vi "GeneratePhaseGPU.vi"() -> ()   [LabVIEW 2019]
uses:
  <vilib>/vision/NI_Vision_Development_Module.lvlib
panel:
  in  "N Iterations":i32
  out "N Pixels":i32
  out "SLM Size":i32
  out "startCuda Return":i32
  in  "CUDA":bool
  out "stopCUDA Return":i32
  out "generatePhase Return":i32
  out "Path to Image File":path
  out "Desired Amplitude":sgl[][](array[numeric])
  in  "Update":bool
  out "Path to CUDA DLL":path
  out "Desired Amplitude":T1(plugin-control)
  in  "Stop":bool
  out "Phase SLM":T1(plugin-control)
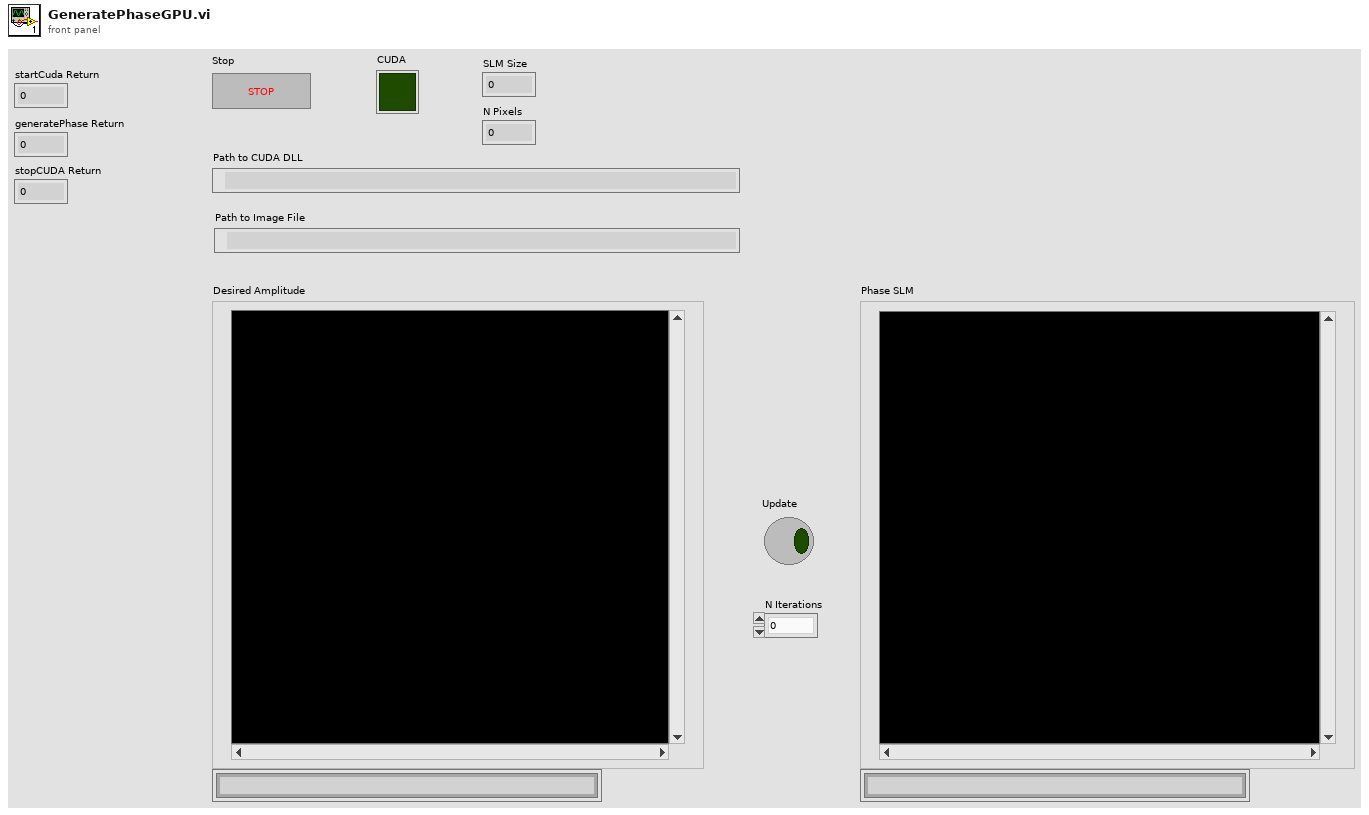
[diagram p1: front panel]
types:
  T1 = typedef "IMAQ Image.ctl" = refnum<image>
  T2 = typedef "Image Type" = u32
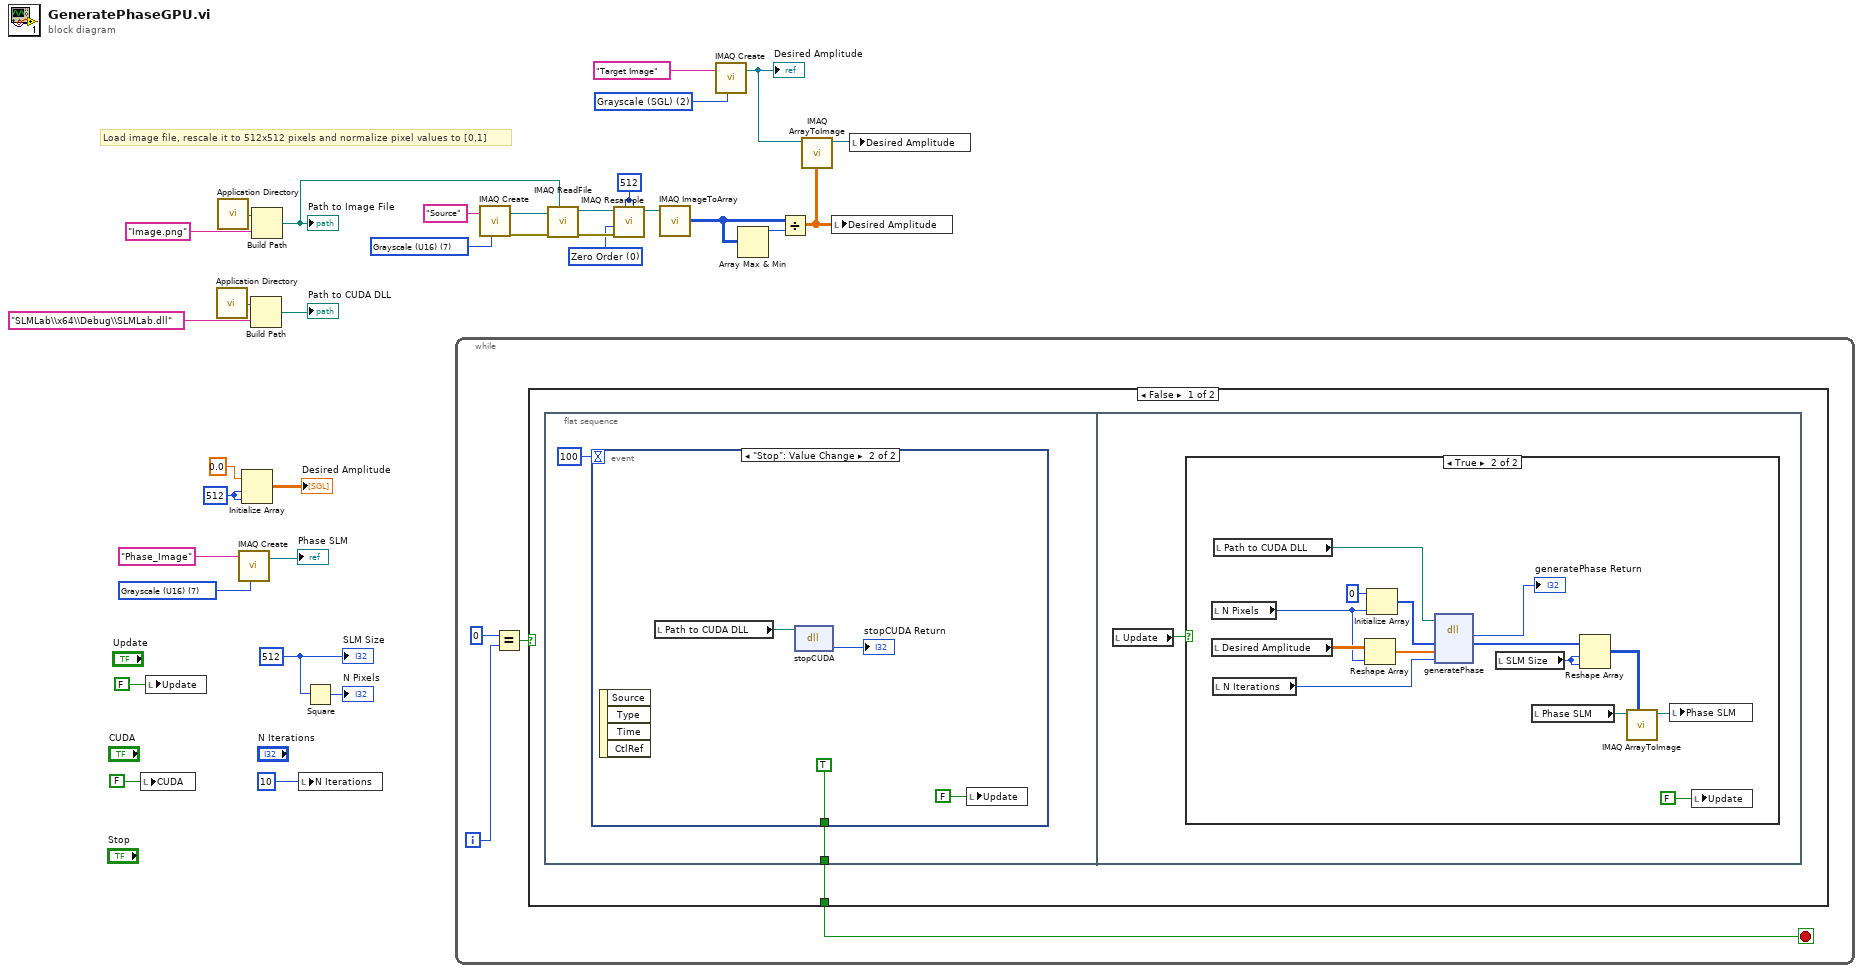
[diagram p0: block diagram]
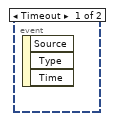
[diagram p2: hidden frame]
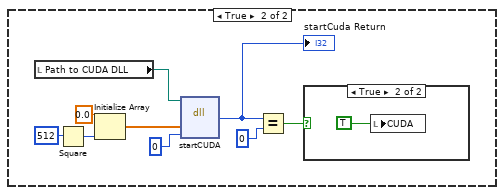
[diagram p4: hidden frame]
diagram:
  w3 = 512
  w16 = T2 7 items=["Grayscale (U8)", "Grayscale (I16)", "Grayscale (SGL)", "Complex (CSG)", "RGB (U32)", "HSL (U32)", "RGB (U64)", "Grayscale (U16)"] ("Image Type")
  w13 = 512
  w12 = u32 0 items=["Zero Order", "Bi-Linear", "Quadratic", "Cubic Spline"] ("Interpolation Type")
  w23 = 512 ("dimension size")
  w29 = T2 2 items=["Grayscale (U8)", "Grayscale (I16)", "Grayscale (SGL)", "Complex (CSG)", "RGB (U32)", "HSL (U32)", "RGB (U64)", "Grayscale (U16)"] ("Image Type")
  w32 = T2 7 items=["Grayscale (U8)", "Grayscale (I16)", "Grayscale (SGL)", "Complex (CSG)", "RGB (U32)", "HSL (U32)", "RGB (U64)", "Grayscale (U16)"] ("Image Type")
  # "Load image file, rescale it to 512x512 pixels and normalize pixel values to [0,1]"
  n1 = local write "CUDA"(FALSE ("Update SLM")) -> ()
  n2 = local write "Update"(FALSE ("Update SLM")) -> ()
  n3 = call <vilib>:"Application Directory.vi"() -> ("Application Directory"=w26:path)
  n4 = call <vilib>:"Application Directory.vi"() -> ("Application Directory"=w8:path)
  n5 = call "IMAQ Create"("Image Name"="Phase_Image", "Image Type"=w32) -> ("New Image"=→"Phase SLM":T1)  [unwired: 3 in, 1 out]
  n6 = Initialize Array(sgl 0.0, w23, w23) -> (→"Desired Amplitude":sgl[][])
  n7 = Build Path(base path=w26, name or relative path="SLMLab\\x64\\Debug\\SLMLab.dll") -> (appended path=→"Path to CUDA DLL":path)
  n8 = Build Path(base path=w8, name or relative path="Image.png") -> (appended path=w5:path)
  "Path to Image File" <- w5
  n9 = local write "N Iterations"(10) -> ()
  n10 = Square(x=w3) -> (x^2=→"N Pixels":i32)
  n11 = while {
    i -> [w35]
    stop <- w34 stop-if-true
    n12 = Equal?(x=0, y=w35) -> (x = y?=w36:bool)
    n13 = case shown="False" w36 {
      tunnel: [w38 _] -> w34
      frame False {
        n14 = flat-sequence {
          tunnel: [w40] -> w38
          frame #0 {
            n15 = event shown="[1] \"Stop\": Value Change" {
              selector: _ -> [_ _]
              dyn-events: _ -> [_ _]
              timeout: 100 -> [_ _]
              tunnel: [_ TRUE] -> w40
              event Timeout {
                n16 = event-data() -> ()  [unwired: 1 in, 3 out]
              }
              event "Stop": Value Change {
                n17 = event-data() -> ()  [unwired: 1 in, 4 out]
                n18 = local read "Path to CUDA DLL"() -> (w42:path)
                n19 = dll-call lib="?" fn="stopCUDA"(path in=w42) -> ("Return Value"=→"stopCUDA Return":i32)  [unwired: 2 in, 2 out]
                n20 = local write "Update"(FALSE ("Update SLM")) -> ()
              }
            }
          }
          frame #1 {
            n21 = local read "Update"() -> (w45:bool)
            n22 = case shown="True" w45 {
              frame False {
              }
              frame True {
                n23 = local read "N Pixels"() -> (w48:i32)
                n24 = local read "Desired Amplitude"() -> (w59:sgl[][])
                n25 = local read "N Iterations"() -> (w46:i32)
                n26 = local read "Path to CUDA DLL"() -> (w50:path)
                n27 = Reshape Array(w59, w48) -> (w58:sgl[])
                n28 = Initialize Array(u16 0 ("element"), w48) -> (w51:u16[])
                n29 = dll-call lib="?" fn="generatePhase"(path in=w50, "h_pSLM_uint16"=w51, "h_dAmplitude"=w58, "n_iterations"=w46) -> ("Return Value"=→"generatePhase Return":i32, "h_pSLM_uint16"=w56:u16[])  [unwired: 4 in, 2 out]
                n30 = local read "SLM Size"() -> (w47:i32)
                n31 = local read "Phase SLM"() -> (w53:T1)
                n32 = Reshape Array(w56, w47, w47) -> (w55:u16[][])
                n33 = call "IMAQ ArrayToImage"("Image Pixels (U16)"=w55, "Image"=w53) -> ("Image Out"=w54:T1)  [unwired: 8 in, 1 out]
                n34 = local write "Phase SLM"(w54) -> ()
                n35 = local write "Update"(FALSE ("Update SLM")) -> ()
              }
            }
          }
        }
      }
      frame True {
        n36 = local read "Path to CUDA DLL"() -> (w63:path)
        n37 = Square(x=512 ("dimension size")) -> (x^2=w66:i32)
        n38 = Initialize Array(sgl 0.0 ("element"), w66) -> (w64:sgl[])
        n39 = dll-call lib="?" fn="startCUDA"(path in=w63, "h_pSLMstart"=w64, "deviceID"=0) -> ("Rückgabetyp"=w62:i32)  [unwired: 4 in, 2 out]
        "startCuda Return" <- w62
        n40 = Equal?(x=w62, y=0) -> (x = y?=w60:bool)
        n41 = case shown="True" w60 {
          frame False {
          }
          frame True {
            n42 = local write "CUDA"(TRUE ("Update SLM")) -> ()
          }
        }
      }
    }
  }
  n43 = call "IMAQ Create"("Image Name"="Source", "Image Type"=w16) -> ("New Image"=w9:T1, "error out"=w10:errorcluster)  [unwired: 3 in]
  n44 = call "IMAQ ReadFile"("File Path"=w5, "error in (no error)"=w10, "Image"=w9) -> ("error out"=w15:errorcluster, "Image Out"=w11:T1)  [unwired: 4 in, 3 out]
  n45 = call "IMAQ Resample"("X Resolution"=w13, "Y Resolution"=w13, "error in (no error)"=w15, "Interpolation Type"=w12, "Image Src"=w11) -> ("Image Dst Out"=w19:T1)  [unwired: 5 in, 1 out]
  n46 = call "IMAQ ImageToArray"("Image"=w19) -> ("Image Pixels (U16)"=w6:u16[][])  [unwired: 3 in, 4 out]
  n47 = call "IMAQ Create"("Image Name"="Target Image", "Image Type"=w29) -> ("New Image"=w1:T1)  [unwired: 3 in, 1 out]
  "Desired Amplitude" <- w1
  n48 = Array Max & Min(array=w6) -> (max value=w17:u16)  [unwired: 3 out]
  n49 = Divide(x=w6, y=w17) -> (x/y=w18:dbl[][])
  n50 = call "IMAQ ArrayToImage"("Image Pixels (Float)"=w18, "Image"=w1) -> ("Image Out"=w20:T1)  [unwired: 8 in, 1 out]
  n51 = local write "Desired Amplitude"(w18) -> ()
  n52 = local write "Desired Amplitude"(w20) -> ()
  "SLM Size" <- w3
